vi "Local Button State Store.vi"(7 "Operation":enum16{"Read", "Write"}(ring), 8 "error in (no error)":errorcluster, 9 "Container State":T3, 10 "Display State In":T1={"Buttons Displayed"=0, "Button States"=[], "Button Size"=0, "Button Style"=enum."Classic", "Active Button"=0, "Force Regen?"=FALSE, "Tip String Ref"=refnum}) -> (0 "error out":errorcluster, 2 "Display State Out":T1={"Buttons Displayed"=0, "Button States"=[], "Button Size"=0, "Button Style"=enum."Classic", "Active Button"=0, "Force Regen?"=FALSE, "Tip String Ref"=refnum}, 3 "Button States":refnum<class "Button.lvclass">[](array[class]))   [LabVIEW 2012, in "Toolbar.xctl"]
doc: "Volatile state storage for toolbar XControles (handles multiple instances of the Toolab by indexing data using the container state)"
uses:
  Toolbar.xctl
  Toolbar State.ctl
  Button_Class/Button.lvclass
  Button_Class/Type Defs/Button Style.ctl
  <vilib>/_xctls/Container State.ctl
  <vilib>/_xctls/XControlSupport.lvlib
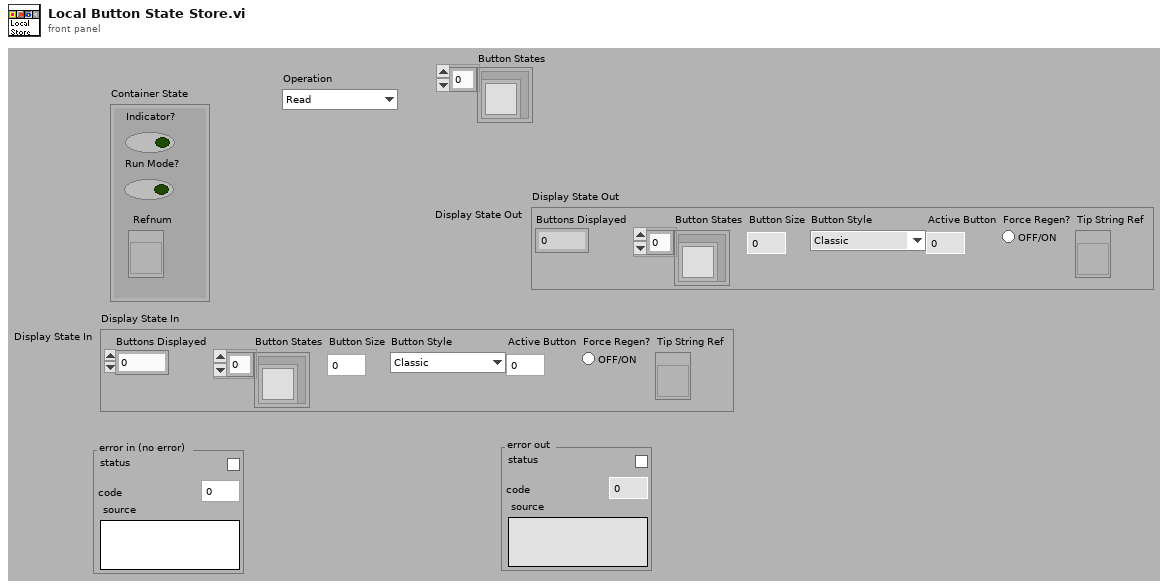
[diagram p1: front panel]
types:
  T1 = typedef "Toolbar.xctl/Toolbar State.ctl" = cluster{"Buttons Displayed":i32, "Button States":refnum<class "Button.lvclass">[], "Button Size":i32, "Button Style":T2, "Active Button":i32, "Force Regen?":bool, "Tip String Ref":refnum<vi>}
  T2 = typedef "Button.lvclass/Button Style.ctl" = enum16{"System", "Modern", "Classic", "Rounded", "Silver", "Ni Theme", "Metallic"}
  T3 = typedef "XControlSupport.lvlib/Container State.ctl" = cluster{"Indicator?":bool, "Run Mode?":bool, " Refnum":refnum<vi>}
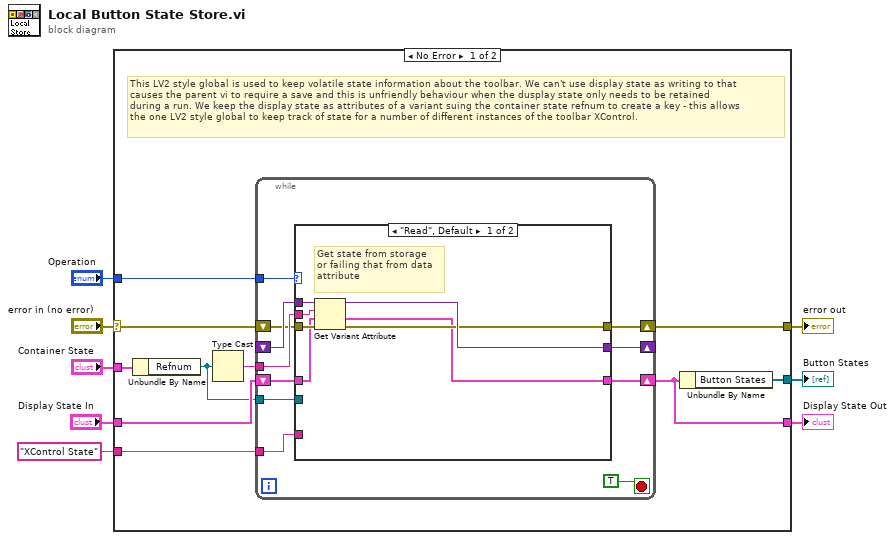
[diagram p0: block diagram]
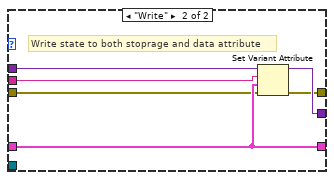
[diagram p2: hidden frame]
diagram:
  n1 = case shown="No Error" "error in (no error)" {
    selector: "error in (no error)" -> [w13 w44]
    tunnel: "Container State" -> [w18 _]
    tunnel: "Operation" -> [w16 _]
    tunnel: "Display State In" -> [w15 w43]
    tunnel: [w12 w44] -> w3
    tunnel: [w10 w43] -> w2
    tunnel: "XControl State" ("name") -> [w11 _]
    tunnel: [w9 _] -> w1
    frame No Error {
      # "This LV2 style global is used to keep volatile state information about the toolbar. We can't use display state as writing to that\ncauses the parent vi to require a save and this is unfriendly behaviour when the dusplay state only needs to be retained\nduring a run. We keep the display state as attributes of a variant suing the container state refnum to create a key - this allows\nthe one LV2 style global to keep track of state for a number of different instances of the toolbar XControl."
      n2 = Unbundle By Name(w18) -> ("Refnum"=w14:refnum<vi>)
      n3 = Type Cast(x=w14) -> (*(type *) &x=w17:string)  [unwired: 1 out]
      n4 = while {
        shift-right: [w28] -> _
        shift-left: _ -> [w29]
        tunnel: w17 -> [w25]
        tunnel: w16 -> [w27]
        tunnel: w14 -> [w24]
        shift-right: [w22] -> w12
        shift-left: w13 -> [w23]
        shift-right: [w21] -> w10
        shift-left: w15 -> [w26]
        tunnel: w11 -> [w19]
        stop <- TRUE stop-if-true
        n5 = case shown="\"Read\", Default" w27 {
          tunnel: w29 -> [w36 w42]
          tunnel: [w35 w41] -> w28
          tunnel: w26 -> [w32 w38]
          tunnel: w25 -> [w34 w40]
          tunnel: w24 -> [_ _]
          tunnel: w23 -> [w33 w37]
          tunnel: [w31 w39] -> w22
          tunnel: [w30 w38] -> w21
          tunnel: w19 -> [_ _]
          frame "Read", Default {
            # "Get state from storage\nor failing that from data\nattribute"
            n6 = Get Variant Attribute(Variant=w36, name=w34, default value (empty Variant)=w32, error in=w33) -> (duplicate Variant=w35:variant, value=w30:T1, error out=w31:errorcluster)  [unwired: 1 out]
          }
          frame "Write" {
            # "Write state to both stoprage and data attribute"
            n7 = Set Variant Attribute(Variant=w42, name=w40, value=w38, error in=w37) -> (Variant out=w41:variant, error out=w39:errorcluster)  [unwired: 1 out]
          }
        }
      }
      n8 = Unbundle By Name(w10) -> ("Button States"=w9:refnum<class "Button.lvclass">[])
    }
    frame Error {
    }
  }
  "error out" <- w3
  "Display State Out" <- w2
  "Button States" <- w1
